vi "Print n Log GD Incoming Msg.vi"(8 "error in (no error)":errorcluster, 9 "Data":variant, 10 "Message":string, 11 "Guardian in":refnum<class "Guardian.lvclass">) -> (0 "error out":errorcluster, 3 "Guardian out":refnum<class "Guardian.lvclass">)   [LabVIEW 2026, in "TALOS.lvlib" / "Guardian.lvlib" / "Guardian.lvclass"]
uses:
  Guardian.lvclass
  C:/LabVIEW Code/TALOS/talos/Ancestor/Ancestor/Ancestor.lvclass
  Ancestor/Ancestor/Ancestor.lvclass/Ancestor.ctl
  Father of all uServices/Father of all uServices/Event Handler Items.ctl
  Classes/uService List/uService List.lvclass/uService List.ctl
  Father of all uServices/Father of all uServices Messages/Event Handler Msg/Event Handler Msg.lvclass/Event Handler Msg.ctl
  <vilib>/Utility/error.llb/Trim Whitespace (string).vi
  Classes/uService List/Get Queue.vi
  Support VIs/Generate Error.vi
  <vilib>/Utility/error.llb/Trim Whitespace One-Sided.vi
  FGV/Error Memory/Get Error Description.vi
  Support VIs/Get PC name.vi
  Support VIs/Get Class Name.vi
  <vilib>/Utility/error.llb/Clear Errors.vi
  FGV/Error Memory/Error Memory Core.vi
  <vilib>/AdvancedString/Delimited String to 1D String Array.vi
  <vilib>/AdvancedString/Delimited String to 1D String Array (string).vi
  Support VIs/Circus Root Path.vi
  FGV/Error Memory/Error Crt Lvl checker.vi
  FGV/Error Memory/Error Memory Core.vi/40c8088d-b597-4017-91af-faa98e00292e.vi
  FGV/Error Memory/Error Memory Core.vi/d4a3ab98-063c-4e44-b43d-fbdcfe6c2be2.vi
  Support VIs/Global Memory.vi
  <vilib>/Utility/LVClass/Get LV Class Name.vi
  Support VIs/Is in Packed Library.vi
  Support VIs/TALOS Root path.vi
  Support VIs/Read CSV worksheet.vi
  Support VIs/Global Constants.vi
  <vilib>/Utility/error.llb/General Error Handler.vi
  <vilib>/Utility/config.llb/Open Config Data.vi
  <vilib>/Utility/config.llb/Get Section Names.vi
  <vilib>/Utility/config.llb/Get Key Names.vi
  <vilib>/Utility/config.llb/Read Key.vi
  <vilib>/Utility/config.llb/Read Key (String).vi
  <vilib>/Utility/config.llb/Close Config Data.vi
  builds/Actor Framework PPL/Actor Framework.lvlibp/1abvi3w/vi.lib/ActorFramework/Message Enqueuer/Enqueue.vi
  Ancestor/Ancestor/Ancestor.lvclass
  <vilib>/Comparison/Equal/Equal Functor/Equal Functor.lvclass
  builds/Actor Framework PPL/Actor Framework.lvlibp/1abvi3w/vi.lib/ActorFramework/Message Enqueuer/Message Enqueuer.lvclass
  Father of all uServices/Father of all uServices Messages/Event Handler Msg/Event Handler Msg.lvclass
  TALOS.lvlib
  Father of all uServices/Father of all uServices/Father of all uServices.lvclass
  Classes/uService List/uService List.lvclass
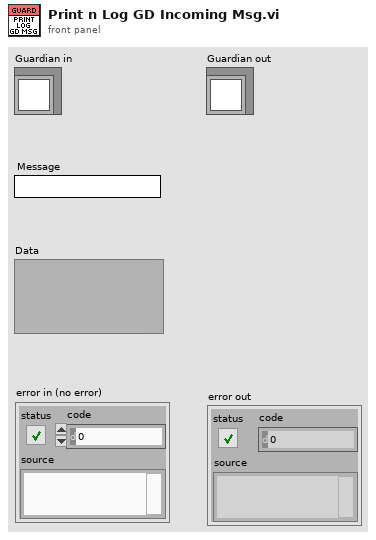
[diagram p1: front panel]
types:
  T1 = typedef "TALOS.lvlib/Father of all uServices.lvlib/Father of all uServices.lvclass/Event Handler Items.ctl" = enum16{"Button Pressed", "Message", "Ready to launch?", "Safe Mode", "Start RUN", "Stop RUN"}
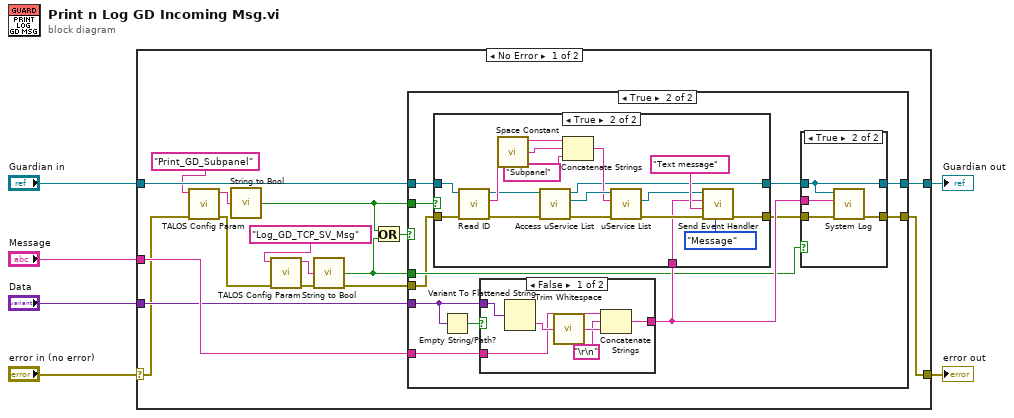
[diagram p0: block diagram]
diagram:
  n1 = case shown="No Error" "error in (no error)" {
    selector: "error in (no error)" -> [w7 w69]
    tunnel: [w16 w68] -> w6
    tunnel: "Guardian in" -> [w13 w68]
    tunnel: [w10 w69] -> w4
    tunnel: "Message" -> [w9 _]
    tunnel: "Data" -> [w8 _]
    frame No Error {
      n2 = call "TALOS Config Param.vi"("error in (no error)"=w7, "Parameter Name"="Print_GD_Subpanel") -> ("error out"=w17:errorcluster, "Output"=w12:string)  [unwired: 8 in]
      n3 = call "String to Bool.vi"("String"=w12) -> ("Boolean"=w21:bool)
      n4 = call "TALOS Config Param.vi"("error in (no error)"=w17, "Parameter Name"="Log_GD_TCP_SV_Msg") -> ("error out"=w18:errorcluster, "Output"=w15:string)  [unwired: 8 in]
      n5 = call "String to Bool.vi"("String"=w15) -> ("Boolean"=w20:bool)
      n6 = Or(x=w21, y=w20) -> (x .or. y?=w19:bool)
      n7 = case shown="True" w19 {
        tunnel: w8 -> [_ w34]
        tunnel: w9 -> [_ w33]
        tunnel: [w22 w32] -> w10
        tunnel: w13 -> [w23 w28]
        tunnel: w21 -> [_ w27]
        tunnel: w20 -> [_ w26]
        tunnel: [w23 w25] -> w16
        tunnel: w18 -> [w22 w24]
        frame False {
        }
        frame True {
          n8 = Empty String/Path?(string/path=w34) -> (empty?=w35:bool)
          n9 = case shown="False" w35 {
            tunnel: w34 -> [w66 _]
            tunnel: w33 -> [w63 w67]
            tunnel: [w61 w67] -> w31
            frame False {
              n10 = Variant To Flattened String(Variant=w66) -> (data string=w65:string)  [unwired: 1 out]
              n11 = call-poly <vilib>:"Trim Whitespace.vi"("string"=w65) -> ("trimmed string"=w64:string)  [unwired: 1 in]
              n12 = Concatenate Strings(w63, "\r\n", w64) -> (w61:string)
            }
            frame True {
            }
          }
          n13 = case shown="True" w27 {
            tunnel: w31 -> [_ w51]
            tunnel: [w37 w44] -> w30
            tunnel: [w36 w43] -> w29
            tunnel: w28 -> [w37 w40]
            tunnel: w24 -> [w36 w39]
            frame False {
            }
            frame True {
              n14 = call "Read ID.vi"("error in (no error)"=w39, "Ancestor in"=w40) -> ("error out"=w38:errorcluster, "ID"=w42:string, "Ancestor out"=w41:refnum<class "Guardian.lvclass">)  [unwired: 7 in]
              n15 = call <vilib>:"Space Constant.vi"() -> ("String"=w45:string)
              n16 = call-dynamic "Access uService List.vi"("error in (no error)"=w38, "Ancestor in"=w41) -> ("error out"=w49:errorcluster, "uService List out"=w48:refnum<class "uService List.lvclass">, "Ancestor out"=w44:refnum<class "Guardian.lvclass">)  [unwired: 7 in]
              n17 = Concatenate Strings(w42, w45, "Subpanel" ("string")) -> (w47:string)
              n18 = call-poly "uService List.vi"("error in (no error)"=w49, "ID"=w47, "uService List in"=w48) -> ("error out"=w54:errorcluster, "uService Queue"=w50:refnum<class "Message Enqueuer.lvclass">)  [unwired: 6 in, 1 out]
              n19 = call "Send Event Handler.vi"("Event type"=Event_Handler_Items."Message", "error in (no error)"=w54, "Item Name"="Text message" ("Message"), "Data"=w51, "Message Enqueuer"=w50) -> ("error out"=w43:errorcluster)  [unwired: 5 in, 1 out]
            }
          }
          n20 = case shown="True" w26 {
            tunnel: [w56 w60] -> w32
            tunnel: w31 -> [_ w59]
            tunnel: w30 -> [w55 w57]
            tunnel: w29 -> [w56 w58]
            tunnel: [w55 w57] -> w25
            frame False {
            }
            frame True {
              n21 = call "System Log.vi"("error in (no error)"=w58, "Text to log"=w59, "Object in"=w57) -> ("error out"=w60:errorcluster)  [unwired: 8 in]
            }
          }
        }
      }
    }
    frame Error {
    }
  }
  "Guardian out" <- w6
  "error out" <- w4
